vi "WPI_CANTalonSRX_Receive.vi"(11 "Device ID (0)":u8) -> (3 "Device ID":u8)   [LabVIEW 2016]
uses:
  <vilib>/Rock Robotics/WPI/ThirdParty/CanMotor/TalonSRX/WPI_CANTalonSRX_MessageIDs.ctl
  <vilib>/Rock Robotics/WPI/ThirdParty/CanMotor/TalonSRX/WPI_CANTalonSRX_GlobalOps.ctl
  <vilib>/Rock Robotics/WPI/ThirdParty/CanMotor/TalonSRX/WPI_CANTalonSRX_GlobalStatus.ctl
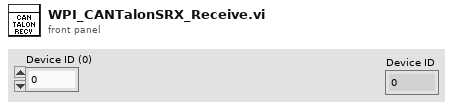
[diagram p1: front panel]
types:
  T1 = typedef "WPI_CANTalonSRX_MessageIDs.ctl" = u32
  T2 = typedef "WPI_CANTalonSRX_GlobalStatus.ctl" = cluster{"Applied Throttle":dbl, "Module Enabled":bool, "CAN Error":errorcluster, "Closed Loop Error":dbl, "Forward Limit Switch Closed":bool, "Reverse Limit Switch Closed":bool, "Sensor Position":dbl, "Sensor Velocity":dbl, "Current":dbl, "Sticky Fault - Over Temp":bool, "Sticky Fault - Under Voltage":bool, "Sticky Fault - Forward Limit":bool, "Sticky Fault - Reverse Limit":bool, "Sticky Fault - Forward Soft Limit":bool, "Sticky Fault - Reverse Soft Limit":bool, "Brake is Enabled":bool, "Encoder Position":dbl, "Encoder Velocity":dbl, "Encoder Index Count":dbl, "Encoder A Pin State":bool, "Encoder B Pin State":bool, "Encoder Index Pin State":bool, "Analog In":dbl, "Analog In Velocity":dbl, "Temperature (C)":dbl, "Battery Voltage":dbl, "Control 5 Is Supported":bool, "Current Profile Slot Select":dbl, "Pos Div 8":bool, "Vel Div 4":bool, "Pulse Width Position":i32, "Pulse Width Velocity":i32, "Pulse Width Rise To Rise (us)":i32, "Pulse Width Rise To Fall (us)":i32, "Mot Prof Active Is Under Run":bool, "Mot Prof Active Has Under Run":bool, "Mot Prof Active Is Last":bool, "Mot Prof Active Velocity Only":bool, "Mot Prof Active Is Valid":bool, "Mot Prof Buffer Is Full":bool, "Mot Prof Active Profile Slot Select":i32, "Mot Prof NextID":i32, "Mot Prof Count":i32, "Mot Prof Active Velocity":dbl, "Mot Prof Active Position":dbl, "Mot Prof Output Enable":i32}
  T3 = typedef "WPI_CANTalonSRX_GlobalOps.ctl" = enum16{"Read For Send", "Write After Receive General", "Write After Receive Feedback", "Write After Receive Encoder", "Write After Receive Ain", "Write Error", "Get All", "Set Output", "Set Mode", "Set Master ID", "Set Brake Mode", "Set Reverse Feedback Sensor", "Set Reverse Closed Loop Output", "Set Override Limits", "Set Forward Limit Enabled", "Set Reverse Limit Enabled", "Set Feedback Select", "Set Profile Select", "Set Throttle Ramp Rate", "Disable", "Set Enc Codes Per Rev", "Set Num Pot Turns", "Set Control Frame Rate", "Enable Legacy Control", "Write After Receive Pulse Width", "Set Enable Frame Rate", "Write After Receive Motion Profile", "Set Motion Profile Flow Control", "Set Motion Profile Control Frame Rate", "Set Current Limit Enable"}
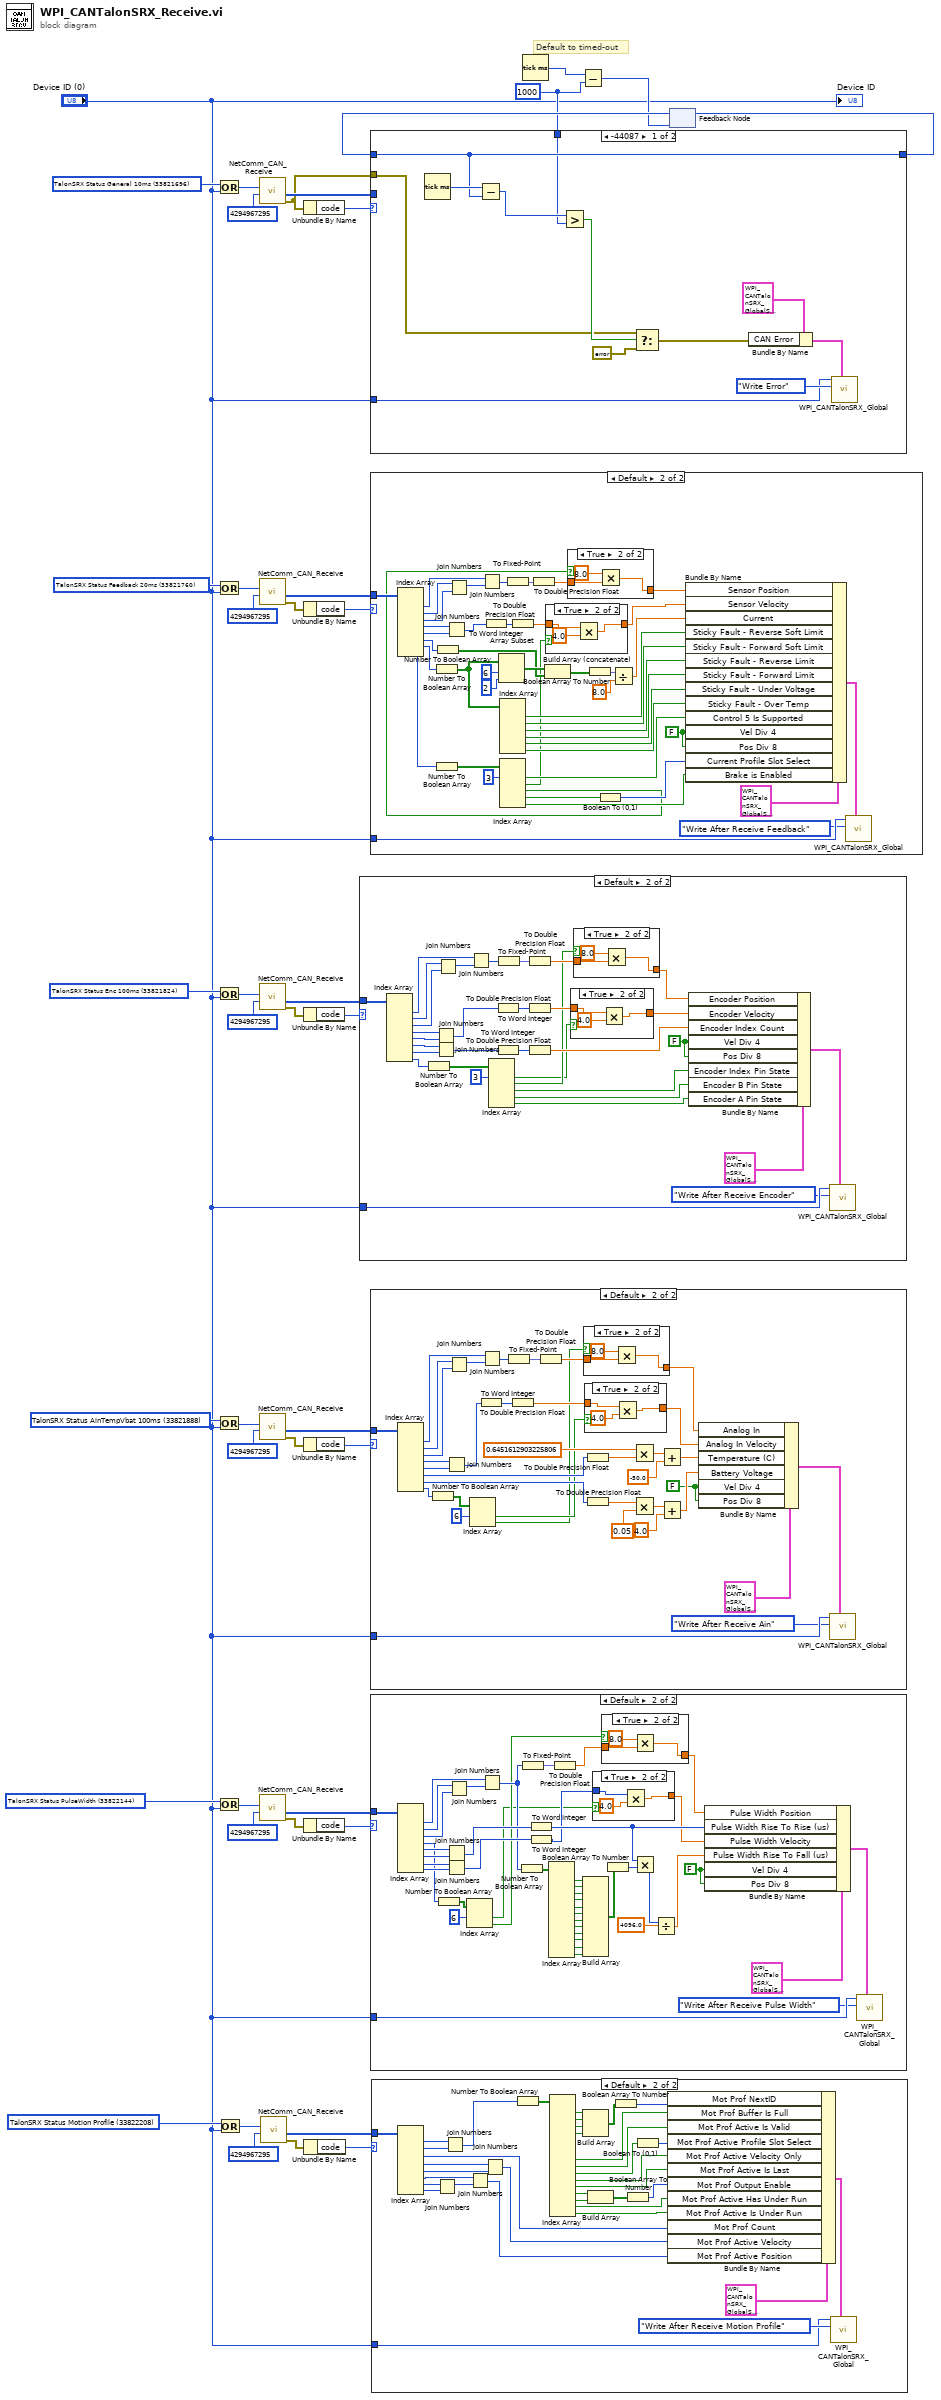
[diagram p0: block diagram]
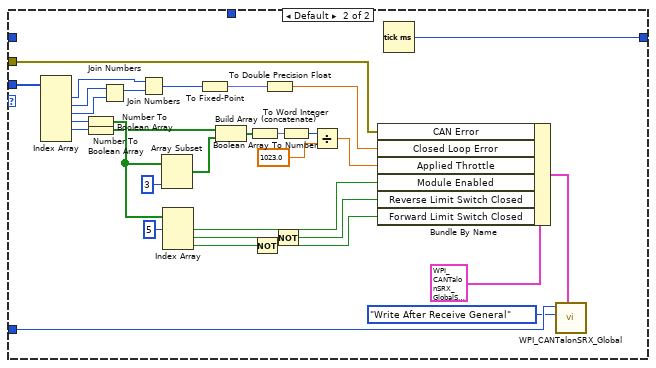
[diagram p15: hidden frame]
diagram:
  w2 = T1 33822208 items=["TalonSRX Control General 10ms"=33816576, "TalonSRX Control Rates Slow"=33816640, "TalonSRX Control ClearFlags Slow"=33816704, "TalonSRX Status General 10ms"=33821696, "TalonSRX Status Feedback 20ms"=33821760, "TalonSRX Status Enc 100ms"=33821824, "TalonSRX Status AinTempVbat 100ms"=33821888, "TalonSRX Status Startup Once"=33821952, "TalonSRX Status Debug"=33822080, "TalonSRX Config SetGainsSlot0 A"=33823808, "TalonSRX Config SetGainsSlot0 B"=33823872, "TalonSRX Config SetGainsSlot1 A"=33823936, "TalonSRX Config SetGainsSlot1 B"=33824000, "TalonSRX Config SetSoftLimits"=33824064, "TalonSRX Config WebControl"=33824128, "TalonSRX Param Request"=33822720, "TalonSRX Param Response"=33822784, "TalonSRX Param Set"=33822848, "TalonSRX Status PulseWidth"=33822144, "TalonSRX Status Motion Profile"=33822208, "TalonSRX Control General 5"=33816832, "TalonSRX Control Motion Profile Add"=33816896] ("Talon SRX Control Frame")
  w8 = T1 33822144 items=["TalonSRX Control General 10ms"=33816576, "TalonSRX Control Rates Slow"=33816640, "TalonSRX Control ClearFlags Slow"=33816704, "TalonSRX Status General 10ms"=33821696, "TalonSRX Status Feedback 20ms"=33821760, "TalonSRX Status Enc 100ms"=33821824, "TalonSRX Status AinTempVbat 100ms"=33821888, "TalonSRX Status Startup Once"=33821952, "TalonSRX Status Debug"=33822080, "TalonSRX Config SetGainsSlot0 A"=33823808, "TalonSRX Config SetGainsSlot0 B"=33823872, "TalonSRX Config SetGainsSlot1 A"=33823936, "TalonSRX Config SetGainsSlot1 B"=33824000, "TalonSRX Config SetSoftLimits"=33824064, "TalonSRX Config WebControl"=33824128, "TalonSRX Param Request"=33822720, "TalonSRX Param Response"=33822784, "TalonSRX Param Set"=33822848, "TalonSRX Status PulseWidth"=33822144, "TalonSRX Status Motion Profile"=33822208, "TalonSRX Control General 5"=33816832, "TalonSRX Control Motion Profile Add"=33816896] ("Talon SRX Control Frame")
  w15 = u32 1000 ("y")
  w21 = T1 33821888 items=["TalonSRX Control General 10ms"=33816576, "TalonSRX Control Rates Slow"=33816640, "TalonSRX Control ClearFlags Slow"=33816704, "TalonSRX Status General 10ms"=33821696, "TalonSRX Status Feedback 20ms"=33821760, "TalonSRX Status Enc 100ms"=33821824, "TalonSRX Status AinTempVbat 100ms"=33821888, "TalonSRX Status Startup Once"=33821952, "TalonSRX Status Debug"=33822080, "TalonSRX Config SetGainsSlot0 A"=33823808, "TalonSRX Config SetGainsSlot0 B"=33823872, "TalonSRX Config SetGainsSlot1 A"=33823936, "TalonSRX Config SetGainsSlot1 B"=33824000, "TalonSRX Config SetSoftLimits"=33824064, "TalonSRX Config WebControl"=33824128, "TalonSRX Param Request"=33822720, "TalonSRX Param Response"=33822784, "TalonSRX Param Set"=33822848]
  w28 = T1 33821824 items=["TalonSRX Control General 10ms"=33816576, "TalonSRX Control Rates Slow"=33816640, "TalonSRX Control ClearFlags Slow"=33816704, "TalonSRX Status General 10ms"=33821696, "TalonSRX Status Feedback 20ms"=33821760, "TalonSRX Status Enc 100ms"=33821824, "TalonSRX Status AinTempVbat 100ms"=33821888, "TalonSRX Status Startup Once"=33821952, "TalonSRX Status Debug"=33822080, "TalonSRX Config SetGainsSlot0 A"=33823808, "TalonSRX Config SetGainsSlot0 B"=33823872, "TalonSRX Config SetGainsSlot1 A"=33823936, "TalonSRX Config SetGainsSlot1 B"=33824000, "TalonSRX Config SetSoftLimits"=33824064, "TalonSRX Config WebControl"=33824128, "TalonSRX Param Request"=33822720, "TalonSRX Param Response"=33822784, "TalonSRX Param Set"=33822848]
  w33 = T1 33821760 items=["TalonSRX Control General 10ms"=33816576, "TalonSRX Control Rates Slow"=33816640, "TalonSRX Control ClearFlags Slow"=33816704, "TalonSRX Status General 10ms"=33821696, "TalonSRX Status Feedback 20ms"=33821760, "TalonSRX Status Enc 100ms"=33821824, "TalonSRX Status AinTempVbat 100ms"=33821888, "TalonSRX Status Startup Once"=33821952, "TalonSRX Status Debug"=33822080, "TalonSRX Config SetGainsSlot0 A"=33823808, "TalonSRX Config SetGainsSlot0 B"=33823872, "TalonSRX Config SetGainsSlot1 A"=33823936, "TalonSRX Config SetGainsSlot1 B"=33824000, "TalonSRX Config SetSoftLimits"=33824064, "TalonSRX Config WebControl"=33824128, "TalonSRX Param Request"=33822720, "TalonSRX Param Response"=33822784, "TalonSRX Param Set"=33822848]
  w40 = T1 33821696 items=["TalonSRX Control General 10ms"=33816576, "TalonSRX Control Rates Slow"=33816640, "TalonSRX Control ClearFlags Slow"=33816704, "TalonSRX Status General 10ms"=33821696, "TalonSRX Status Feedback 20ms"=33821760, "TalonSRX Status Enc 100ms"=33821824, "TalonSRX Status AinTempVbat 100ms"=33821888, "TalonSRX Status Startup Once"=33821952, "TalonSRX Status Debug"=33822080, "TalonSRX Config SetGainsSlot0 A"=33823808, "TalonSRX Config SetGainsSlot0 B"=33823872, "TalonSRX Config SetGainsSlot1 A"=33823936, "TalonSRX Config SetGainsSlot1 B"=33824000, "TalonSRX Config SetSoftLimits"=33824064, "TalonSRX Config WebControl"=33824128, "TalonSRX Param Request"=33822720, "TalonSRX Param Response"=33822784, "TalonSRX Param Set"=33822848]
  # "Default to timed-out"
  n1 = Or(x=w40, y="Device ID (0)") -> (x .or. y?=w41:T1)
  n2 = Or(x=w33, y="Device ID (0)") -> (x .or. y?=w32:T1)
  n3 = Or(x=w28, y="Device ID (0)") -> (x .or. y?=w29:T1)
  n4 = Or(x=w21, y="Device ID (0)") -> (x .or. y?=w20:T1)
  n5 = Or(x=w8, y="Device ID (0)") -> (x .or. y?=w12:T1)
  n6 = Or(x=w2, y="Device ID (0)") -> (x .or. y?=w6:T1)
  n7 = call <vilib>:"NetComm_CAN_Receive.vi"("Message ID Mask"=u32 4294967295, "Message ID"=w41) -> ("error out"=w38:errorcluster, "Data"=w42:u8[])  [unwired: 6 in, 2 out]
  n8 = call <vilib>:"NetComm_CAN_Receive.vi"("Message ID Mask"=u32 4294967295, "Message ID"=w32) -> ("error out"=w35:errorcluster, "Data"=w31:u8[])  [unwired: 6 in, 2 out]
  n9 = call <vilib>:"NetComm_CAN_Receive.vi"("Message ID Mask"=u32 4294967295, "Message ID"=w29) -> ("error out"=w26:errorcluster, "Data"=w30:u8[])  [unwired: 6 in, 2 out]
  n10 = call <vilib>:"NetComm_CAN_Receive.vi"("Message ID Mask"=u32 4294967295, "Message ID"=w20) -> ("error out"=w23:errorcluster, "Data"=w19:u8[])  [unwired: 6 in, 2 out]
  n11 = call <vilib>:"NetComm_CAN_Receive.vi"("Message ID Mask"=u32 4294967295, "Message ID"=w12) -> ("error out"=w10:errorcluster, "Data"=w13:u8[])  [unwired: 6 in, 2 out]
  n12 = call <vilib>:"NetComm_CAN_Receive.vi"("Message ID Mask"=u32 4294967295, "Message ID"=w6) -> ("error out"=w4:errorcluster, "Data"=w7:u8[])  [unwired: 6 in, 2 out]
  n13 = Unbundle By Name(w38) -> ("code"=w37:i32)
  n14 = Unbundle By Name(w35) -> ("code"=w36:i32)
  n15 = Unbundle By Name(w26) -> ("code"=w25:i32)
  n16 = Unbundle By Name(w23) -> ("code"=w24:i32)
  n17 = Unbundle By Name(w10) -> ("code"=w9:i32)
  n18 = Unbundle By Name(w4) -> ("code"=w3:i32)
  n19 = case shown="Default" w25 {
    tunnel: "Device ID (0)" -> [_ w75]
    tunnel: w30 -> [_ w74]
    frame -44087 {
    }
    frame Default {
      w43 = FALSE ("Vel Div 4")
      n20 = Index Array(array=w74) -> (element #1=w67:u8, element #2=w69:u8, element #3=w66:u8, element #4=w65:u8, element #5=w64:u8, element #6=w60:u8, element #7=w59:u8, element #8=w62:u8)  [unwired: 8 in]
      n21 = Number To Boolean Array(number=w62) -> (Boolean array=w72:bool[])
      n22 = Join Numbers(hi=w65, lo=w64) -> ((hi.lo)=w63:u16)
      n23 = Join Numbers(hi=w60, lo=w59) -> ((hi.lo)=w56:u16)
      n24 = Join Numbers(hi=w69, lo=w66) -> ((hi.lo)=w68:u16)
      n25 = Join Numbers(hi=w67, lo=w68) -> ((hi.lo)=w54:u32)
      n26 = Index Array(array=w72, index #1=3 ("index")) -> (element #1=w44:bool, element #2=w45:bool, element #3=w46:bool, element #4=w47:bool, element #5=w48:bool)  [unwired: 4 in]
      n27 = To Word Integer(number=w63) -> (16bit integer=w57:i16)
      n28 = To Word Integer(number=w56) -> (16bit integer=w55:i16)
      n29 = To Fixed-Point(number=w54) -> (fixed-point=w53:fxp<+/-,24,24>)  [unwired: 1 in]
      n30 = To Double Precision Float(number=w53) -> (double precision float=w51:dbl)
      n31 = To Double Precision Float(number=w57) -> (double precision float=w52:dbl)
      n32 = To Double Precision Float(number=w55) -> (double precision float=w61:dbl)
      n33 = case shown="True" w44 {
        tunnel: w52 -> [w76 w79]
        tunnel: [w76 w77] -> w50
        frame False {
        }
        frame True {
          n34 = Multiply(x=w79, y=4.0) -> (x*y=w77:dbl)
        }
      }
      n35 = case shown="True" w45 {
        tunnel: w51 -> [w80 w83]
        tunnel: [w80 w81] -> w49
        frame False {
        }
        frame True {
          n36 = Multiply(x=8.0, y=w83) -> (x*y=w81:dbl)
        }
      }
      n37 = Bundle By Name(cluster=T2 {"Applied Throttle"=0.0, "Module Enabled"=FALSE, "CAN Error"={"status"=FALSE, "code"=0, "source"=""}, "Closed Loop Error"=0.0, "Forward Limit Switch Closed"=FALSE, "Reverse Limit Switch Closed"=FALSE, "Sensor Position"=0.0, "Sensor Velocity"=0.0, "Current"=0.0, "Sticky Fault - Over Temp"=FALSE, "Sticky Fault - Under Voltage"=FALSE, "Sticky Fault - Forward Limit"=FALSE, "Sticky Fault - Reverse Limit"=FALSE, "Sticky Fault - Forward Soft Limit"=FALSE, "Sticky Fault - Reverse Soft Limit"=FALSE, "Brake is Enabled"=FALSE, "Encoder Position"=0.0, "Encoder Velocity"=0.0, "Encoder Index Count"=0.0, "Encoder A Pin State"=FALSE, "Encoder B Pin State"=FALSE, "Encoder Index Pin State"=FALSE, "Analog In"=0.0, "Analog In Velocity"=0.0, "Temperature (C)"=0.0, "Battery Voltage"=0.0, "Control 5 Is Supported"=FALSE, "Current Profile Slot Select"=0.0, "Pos Div 8"=FALSE, "Vel Div 4"=FALSE, "Pulse Width Position"=0, "Pulse Width Velocity"=0, "Pulse Width Rise To Rise (us)"=0, "Pulse Width Rise To Fall (us)"=0, "Mot Prof Active Is Under Run"=FALSE, "Mot Prof Active Has Under Run"=FALSE, "Mot Prof Active Is Last"=FALSE, "Mot Prof Active Velocity Only"=FALSE, "Mot Prof Active Is Valid"=FALSE, "Mot Prof Buffer Is Full"=FALSE, "Mot Prof Active Profile Slot Select"=0, "Mot Prof NextID"=0, "Mot Prof Count"=0, "Mot Prof Active Velocity"=0.0, "Mot Prof Active Position"=0.0, "Mot Prof Output Enable"=0} ("Write After Receive"), "Encoder Position"=w49, "Encoder Velocity"=w50, "Encoder Index Count"=w61, "Vel Div 4"=w43, "Pos Div 8"=w43, "Encoder Index Pin State"=w46, "Encoder B Pin State"=w47, "Encoder A Pin State"=w48) -> (w73:T2)
      n38 = call <vilib>:"WPI_CANTalonSRX_Global.vi"("Write After Receive"=w73, "Operation"=WPI_CANTalonSRX_GlobalOps."Write After Receive Encoder", "Device ID (0)"=w75) -> ()  [unwired: 6 in, 3 out]
    }
  }
  n39 = case shown="Default" w36 {
    tunnel: "Device ID (0)" -> [_ w129]
    tunnel: w31 -> [_ w128]
    frame -44087 {
    }
    frame Default {
      w84 = FALSE ("Vel Div 4")
      n40 = Index Array(array=w128) -> (element #1=w117:u8, element #2=w119:u8, element #3=w116:u8, element #4=w115:u8, element #5=w114:u8, element #6=w112:u8, element #7=w111:u8, element #8=w107:u8)  [unwired: 8 in]
      n41 = Number To Boolean Array(number=w111) -> (Boolean array=w126:bool[])
      n42 = Number To Boolean Array(number=w107) -> (Boolean array=w106:bool[])
      n43 = Number To Boolean Array(number=w112) -> (Boolean array=w97:bool[])
      n44 = Join Numbers(hi=w115, lo=w114) -> ((hi.lo)=w113:u16)
      n45 = Join Numbers(hi=w119, lo=w116) -> ((hi.lo)=w118:u16)
      n46 = Join Numbers(hi=w117, lo=w118) -> ((hi.lo)=w96:u32)
      n47 = To Word Integer(number=w113) -> (16bit integer=w99:i16)
      n48 = Array Subset(array=w126, index=6, length=2) -> (w98:bool[])
      n49 = Index Array(array=w126) -> (element #1=w104:bool, element #2=w103:bool, element #3=w102:bool, element #4=w101:bool, element #5=w100:bool, element #6=w105:bool)  [unwired: 6 in]
      n50 = Index Array(array=w106, index #1=3 ("index")) -> (element #1=w93:bool, element #2=w85:bool, element #3=w88:bool, element #4=w91:bool, element #5=w94:bool)  [unwired: 4 in]
      n51 = To Fixed-Point(number=w96) -> (fixed-point=w95:fxp<+/-,24,24>)  [unwired: 1 in]
      n52 = To Double Precision Float(number=w99) -> (double precision float=w87:dbl)
      n53 = To Double Precision Float(number=w95) -> (double precision float=w90:dbl)
      n54 = Build Array (concatenate)(w98, w97) -> (w124:bool[])
      n55 = case shown="True" w85 {
        tunnel: w87 -> [w130 w133]
        tunnel: [w130 w131] -> w86
        frame False {
        }
        frame True {
          n56 = Multiply(x=w133, y=4.0) -> (x*y=w131:dbl)
        }
      }
      n57 = case shown="True" w88 {
        tunnel: w90 -> [w134 w137]
        tunnel: [w134 w135] -> w89
        frame False {
        }
        frame True {
          n58 = Multiply(x=8.0, y=w137) -> (x*y=w135:dbl)
        }
      }
      n59 = Boolean Array To Number(Boolean array=w124) -> (number=w123:fxp<+/-,11,11>)
      n60 = Boolean To (0,1)(Boolean=w91) -> (0, 1=w92:i16)
      n61 = Divide(x=w123, y=8.0) -> (x/y=w109:dbl)
      n62 = Bundle By Name(cluster=T2 {"Applied Throttle"=0.0, "Module Enabled"=FALSE, "CAN Error"={"status"=FALSE, "code"=0, "source"=""}, "Closed Loop Error"=0.0, "Forward Limit Switch Closed"=FALSE, "Reverse Limit Switch Closed"=FALSE, "Sensor Position"=0.0, "Sensor Velocity"=0.0, "Current"=0.0, "Sticky Fault - Over Temp"=FALSE, "Sticky Fault - Under Voltage"=FALSE, "Sticky Fault - Forward Limit"=FALSE, "Sticky Fault - Reverse Limit"=FALSE, "Sticky Fault - Forward Soft Limit"=FALSE, "Sticky Fault - Reverse Soft Limit"=FALSE, "Brake is Enabled"=FALSE, "Encoder Position"=0.0, "Encoder Velocity"=0.0, "Encoder Index Count"=0.0, "Encoder A Pin State"=FALSE, "Encoder B Pin State"=FALSE, "Encoder Index Pin State"=FALSE, "Analog In"=0.0, "Analog In Velocity"=0.0, "Temperature (C)"=0.0, "Battery Voltage"=0.0, "Control 5 Is Supported"=FALSE, "Current Profile Slot Select"=0.0, "Pos Div 8"=FALSE, "Vel Div 4"=FALSE, "Pulse Width Position"=0, "Pulse Width Velocity"=0, "Pulse Width Rise To Rise (us)"=0, "Pulse Width Rise To Fall (us)"=0, "Mot Prof Active Is Under Run"=FALSE, "Mot Prof Active Has Under Run"=FALSE, "Mot Prof Active Is Last"=FALSE, "Mot Prof Active Velocity Only"=FALSE, "Mot Prof Active Is Valid"=FALSE, "Mot Prof Buffer Is Full"=FALSE, "Mot Prof Active Profile Slot Select"=0, "Mot Prof NextID"=0, "Mot Prof Count"=0, "Mot Prof Active Velocity"=0.0, "Mot Prof Active Position"=0.0, "Mot Prof Output Enable"=0} ("Write After Receive"), "Sensor Position"=w89, "Sensor Velocity"=w86, "Current"=w109, "Sticky Fault - Reverse Soft Limit"=w104, "Sticky Fault - Forward Soft Limit"=w103, "Sticky Fault - Reverse Limit"=w102, "Sticky Fault - Forward Limit"=w101, "Sticky Fault - Under Voltage"=w100, "Sticky Fault - Over Temp"=w105, "Control 5 Is Supported"=w93, "Vel Div 4"=w84, "Pos Div 8"=w84, "Current Profile Slot Select"=w92, "Brake is Enabled"=w94) -> (w127:T2)
      n63 = call <vilib>:"WPI_CANTalonSRX_Global.vi"("Write After Receive"=w127, "Operation"=WPI_CANTalonSRX_GlobalOps."Write After Receive Feedback", "Device ID (0)"=w129) -> ()  [unwired: 6 in, 3 out]
    }
  }
  n64 = case shown="Default" w24 {
    tunnel: "Device ID (0)" -> [_ w174]
    tunnel: w19 -> [_ w173]
    frame -44087 {
    }
    frame Default {
      w138 = FALSE ("Vel Div 4")
      n65 = Index Array(array=w173) -> (element #1=w167:u8, element #2=w169:u8, element #3=w166:u8, element #4=w165:u8, element #5=w164:u8, element #6=w160:u8, element #7=w161:u8, element #8=w147:u8)  [unwired: 8 in]
      n66 = Number To Boolean Array(number=w147) -> (Boolean array=w146:bool[])
      n67 = Join Numbers(hi=w165, lo=w164) -> ((hi.lo)=w163:u16)
      n68 = Join Numbers(hi=w169, lo=w166) -> ((hi.lo)=w168:u16)
      n69 = Index Array(array=w146, index #1=6 ("index")) -> (element #1=w140:bool, element #2=w139:bool)  [unwired: 1 in]
      n70 = To Word Integer(number=w163) -> (16bit integer=w150:i16)
      n71 = Join Numbers(hi=w167, lo=w168) -> ((hi.lo)=w149:u32)
      n72 = To Fixed-Point(number=w149) -> (fixed-point=w148:fxp<+/-,24,24>)  [unwired: 1 in]
      n73 = To Double Precision Float(number=w150) -> (double precision float=w142:dbl)
      n74 = To Double Precision Float(number=w148) -> (double precision float=w144:dbl)
      n75 = case shown="True" w139 {
        tunnel: w144 -> [w179 w182]
        tunnel: [w179 w180] -> w143
        frame False {
        }
        frame True {
          n76 = Multiply(x=8.0, y=w182) -> (x*y=w180:dbl)
        }
      }
      n77 = case shown="True" w140 {
        tunnel: w142 -> [w175 w178]
        tunnel: [w175 w176] -> w141
        frame False {
        }
        frame True {
          n78 = Multiply(x=w178, y=4.0) -> (x*y=w176:dbl)
        }
      }
      n79 = To Double Precision Float(number=w160) -> (double precision float=w151:dbl)
      n80 = To Double Precision Float(number=w161) -> (double precision float=w162:dbl)
      n81 = Multiply(x=0.6451612903225806, y=w151) -> (x*y=w155:dbl)
      n82 = Multiply(x=w162, y=0.05 ("x")) -> (x*y=w157:dbl)
      n83 = Add(x=w155, y=-50.0 ("x")) -> (x+y=w153:dbl)
      n84 = Add(x=w157, y=4.0 ("x")) -> (x+y=w159:dbl)
      n85 = Bundle By Name(cluster=T2 {"Applied Throttle"=0.0, "Module Enabled"=FALSE, "CAN Error"={"status"=FALSE, "code"=0, "source"=""}, "Closed Loop Error"=0.0, "Forward Limit Switch Closed"=FALSE, "Reverse Limit Switch Closed"=FALSE, "Sensor Position"=0.0, "Sensor Velocity"=0.0, "Current"=0.0, "Sticky Fault - Over Temp"=FALSE, "Sticky Fault - Under Voltage"=FALSE, "Sticky Fault - Forward Limit"=FALSE, "Sticky Fault - Reverse Limit"=FALSE, "Sticky Fault - Forward Soft Limit"=FALSE, "Sticky Fault - Reverse Soft Limit"=FALSE, "Brake is Enabled"=FALSE, "Encoder Position"=0.0, "Encoder Velocity"=0.0, "Encoder Index Count"=0.0, "Encoder A Pin State"=FALSE, "Encoder B Pin State"=FALSE, "Encoder Index Pin State"=FALSE, "Analog In"=0.0, "Analog In Velocity"=0.0, "Temperature (C)"=0.0, "Battery Voltage"=0.0, "Control 5 Is Supported"=FALSE, "Current Profile Slot Select"=0.0, "Pos Div 8"=FALSE, "Vel Div 4"=FALSE, "Pulse Width Position"=0, "Pulse Width Velocity"=0, "Pulse Width Rise To Rise (us)"=0, "Pulse Width Rise To Fall (us)"=0, "Mot Prof Active Is Under Run"=FALSE, "Mot Prof Active Has Under Run"=FALSE, "Mot Prof Active Is Last"=FALSE, "Mot Prof Active Velocity Only"=FALSE, "Mot Prof Active Is Valid"=FALSE, "Mot Prof Buffer Is Full"=FALSE, "Mot Prof Active Profile Slot Select"=0, "Mot Prof NextID"=0, "Mot Prof Count"=0, "Mot Prof Active Velocity"=0.0, "Mot Prof Active Position"=0.0, "Mot Prof Output Enable"=0} ("Write After Receive"), "Analog In"=w143, "Analog In Velocity"=w141, "Temperature (C)"=w153, "Battery Voltage"=w159, "Vel Div 4"=w138, "Pos Div 8"=w138) -> (w172:T2)
      n86 = call <vilib>:"WPI_CANTalonSRX_Global.vi"("Write After Receive"=w172, "Operation"=WPI_CANTalonSRX_GlobalOps."Write After Receive Ain", "Device ID (0)"=w174) -> ()  [unwired: 6 in, 3 out]
    }
  }
  n87 = case shown="Default" w9 {
    tunnel: "Device ID (0)" -> [_ w228]
    tunnel: w13 -> [_ w227]
    frame -44087 {
    }
    frame Default {
      w183 = FALSE ("Vel Div 4")
      n88 = Index Array(array=w227) -> (element #1=w221:u8, element #2=w223:u8, element #3=w220:u8, element #4=w192:u8, element #5=w216:u8, element #6=w215:u8, element #7=w214:u8, element #8=w213:u8)  [unwired: 8 in]
      n89 = Number To Boolean Array(number=w192) -> (Boolean array=w191:bool[])
      n90 = Join Numbers(hi=w216, lo=w215) -> ((hi.lo)=w219:u16)
      n91 = Join Numbers(hi=w214, lo=w213) -> ((hi.lo)=w218:u16)
      n92 = Join Numbers(hi=w223, lo=w220) -> ((hi.lo)=w222:u16)
      n93 = Index Array(array=w191, index #1=6 ("index")) -> (element #1=w184:bool, element #2=w185:bool)  [unwired: 1 in]
      n94 = Join Numbers(hi=w221, lo=w222) -> ((hi.lo)=w193:u32)
      n95 = Number To Boolean Array(number=w193) -> (Boolean array=w208:bool[])
      n96 = To Fixed-Point(number=w193) -> (fixed-point=w217:fxp<+/-,24,24>)  [unwired: 1 in]
      n97 = To Word Integer(number=w219) -> (16bit integer=w209:i16)
      n98 = To Word Integer(number=w218) -> (16bit integer=w187:i16)
      n99 = Index Array(array=w208) -> (element #1=w198:bool, element #2=w199:bool, element #3=w200:bool, element #4=w201:bool, element #5=w202:bool, element #6=w203:bool, element #7=w204:bool, element #8=w205:bool, element #9=w206:bool, element #10=w207:bool, element #11=w195:bool, element #12=w194:bool)  [unwired: 12 in]
      n100 = To Double Precision Float(number=w217) -> (double precision float=w188:dbl)
      n101 = Build Array(w198, w199, w200, w201, w202, w203, w204, w205, w206, w207, w195, w194) -> (w197:bool[])
      n102 = case shown="True" w184 {
        tunnel: w187 -> [w229 w232]
        tunnel: [w229 w230] -> w186
        frame False {
        }
        frame True {
          n103 = Multiply(x=w232, y=4.0) -> (x*y=w230:dbl)
        }
      }
      n104 = case shown="True" w185 {
        tunnel: w188 -> [w233 w236]
        tunnel: [w233 w234] -> w189
        frame False {
        }
        frame True {
          n105 = Multiply(x=8.0, y=w236) -> (x*y=w234:dbl)
        }
      }
      n106 = Boolean Array To Number(Boolean array=w197) -> (number=w196:u32)
      n107 = Multiply(x=w209, y=w196) -> (x*y=w211:u32)
      n108 = Divide(x=w211, y=4096.0) -> (x/y=w210:dbl)
      n109 = Bundle By Name(cluster=T2 {"Applied Throttle"=0.0, "Module Enabled"=FALSE, "CAN Error"={"status"=FALSE, "code"=0, "source"=""}, "Closed Loop Error"=0.0, "Forward Limit Switch Closed"=FALSE, "Reverse Limit Switch Closed"=FALSE, "Sensor Position"=0.0, "Sensor Velocity"=0.0, "Current"=0.0, "Sticky Fault - Over Temp"=FALSE, "Sticky Fault - Under Voltage"=FALSE, "Sticky Fault - Forward Limit"=FALSE, "Sticky Fault - Reverse Limit"=FALSE, "Sticky Fault - Forward Soft Limit"=FALSE, "Sticky Fault - Reverse Soft Limit"=FALSE, "Brake is Enabled"=FALSE, "Encoder Position"=0.0, "Encoder Velocity"=0.0, "Encoder Index Count"=0.0, "Encoder A Pin State"=FALSE, "Encoder B Pin State"=FALSE, "Encoder Index Pin State"=FALSE, "Analog In"=0.0, "Analog In Velocity"=0.0, "Temperature (C)"=0.0, "Battery Voltage"=0.0, "Control 5 Is Supported"=FALSE, "Current Profile Slot Select"=0.0, "Pos Div 8"=FALSE, "Vel Div 4"=FALSE, "Pulse Width Position"=0, "Pulse Width Velocity"=0, "Pulse Width Rise To Rise (us)"=0, "Pulse Width Rise To Fall (us)"=0, "Mot Prof Active Is Under Run"=FALSE, "Mot Prof Active Has Under Run"=FALSE, "Mot Prof Active Is Last"=FALSE, "Mot Prof Active Velocity Only"=FALSE, "Mot Prof Active Is Valid"=FALSE, "Mot Prof Buffer Is Full"=FALSE, "Mot Prof Active Profile Slot Select"=0, "Mot Prof NextID"=0, "Mot Prof Count"=0, "Mot Prof Active Velocity"=0.0, "Mot Prof Active Position"=0.0, "Mot Prof Output Enable"=0} ("Write After Receive"), "Pulse Width Position"=w189, "Pulse Width Rise To Rise (us)"=w209, "Pulse Width Velocity"=w186, "Pulse Width Rise To Fall (us)"=w210, "Vel Div 4"=w183, "Pos Div 8"=w183) -> (w226:T2)
      n110 = call <vilib>:"WPI_CANTalonSRX_Global.vi"("Write After Receive"=w226, "Operation"=WPI_CANTalonSRX_GlobalOps."Write After Receive Pulse Width", "Device ID (0)"=w228) -> ()  [unwired: 6 in, 3 out]
    }
  }
  n111 = case shown="Default" w3 {
    tunnel: w7 -> [_ w272]
    tunnel: "Device ID (0)" -> [_ w267]
    frame -44087 {
    }
    frame Default {
      n112 = Index Array(array=w272) -> (element #1=w260:u8, element #2=w259:u8, element #3=w237:u8, element #4=w262:u8, element #5=w263:u8, element #6=w266:u8, element #7=w265:u8, element #8=w264:u8)  [unwired: 8 in]
      n113 = Join Numbers(hi=w265, lo=w264) -> ((hi.lo)=w268:u16)
      n114 = Join Numbers(hi=w260, lo=w259) -> ((hi.lo)=w258:u16)
      n115 = Join Numbers(hi=w266, lo=w268) -> ((hi.lo)=w239:u32)
      n116 = Join Numbers(hi=w262, lo=w263) -> ((hi.lo)=w238:u16)
      n117 = Number To Boolean Array(number=w258) -> (Boolean array=w261:bool[])
      n118 = Index Array(array=w261) -> (element #1=w257:bool, element #2=w256:bool, element #3=w255:bool, element #4=w254:bool, element #8=w251:bool, element #9=w250:bool, element #10=w240:bool, element #11=w249:bool, element #12=w248:bool, element #13=w245:bool, element #14=w244:bool, element #15=w246:bool, element #16=w247:bool)  [unwired: 16 in, 3 out]
      n119 = Build Array(w257, w256, w255, w254) -> (w253:bool[])
      n120 = Build Array(w245, w244) -> (w242:bool[])
      n121 = Boolean Array To Number(Boolean array=w253) -> (number=w252:u32)
      n122 = Boolean Array To Number(Boolean array=w242) -> (number=w243:u32)
      n123 = Boolean To (0,1)(Boolean=w240) -> (0, 1=w241:i16)
      n124 = Bundle By Name(cluster=T2 {"Applied Throttle"=0.0, "Module Enabled"=FALSE, "CAN Error"={"status"=FALSE, "code"=0, "source"=""}, "Closed Loop Error"=0.0, "Forward Limit Switch Closed"=FALSE, "Reverse Limit Switch Closed"=FALSE, "Sensor Position"=0.0, "Sensor Velocity"=0.0, "Current"=0.0, "Sticky Fault - Over Temp"=FALSE, "Sticky Fault - Under Voltage"=FALSE, "Sticky Fault - Forward Limit"=FALSE, "Sticky Fault - Reverse Limit"=FALSE, "Sticky Fault - Forward Soft Limit"=FALSE, "Sticky Fault - Reverse Soft Limit"=FALSE, "Brake is Enabled"=FALSE, "Encoder Position"=0.0, "Encoder Velocity"=0.0, "Encoder Index Count"=0.0, "Encoder A Pin State"=FALSE, "Encoder B Pin State"=FALSE, "Encoder Index Pin State"=FALSE, "Analog In"=0.0, "Analog In Velocity"=0.0, "Temperature (C)"=0.0, "Battery Voltage"=0.0, "Control 5 Is Supported"=FALSE, "Current Profile Slot Select"=0.0, "Pos Div 8"=FALSE, "Vel Div 4"=FALSE, "Pulse Width Position"=0, "Pulse Width Velocity"=0, "Pulse Width Rise To Rise (us)"=0, "Pulse Width Rise To Fall (us)"=0, "Mot Prof Active Is Under Run"=FALSE, "Mot Prof Active Has Under Run"=FALSE, "Mot Prof Active Is Last"=FALSE, "Mot Prof Active Velocity Only"=FALSE, "Mot Prof Active Is Valid"=FALSE, "Mot Prof Buffer Is Full"=FALSE, "Mot Prof Active Profile Slot Select"=0, "Mot Prof NextID"=0, "Mot Prof Count"=0, "Mot Prof Active Velocity"=0.0, "Mot Prof Active Position"=0.0, "Mot Prof Output Enable"=0} ("Write After Receive"), "Mot Prof NextID"=w252, "Mot Prof Buffer Is Full"=w251, "Mot Prof Active Is Valid"=w250, "Mot Prof Active Profile Slot Select"=w241, "Mot Prof Active Velocity Only"=w249, "Mot Prof Active Is Last"=w248, "Mot Prof Output Enable"=w243, "Mot Prof Active Has Under Run"=w246, "Mot Prof Active Is Under Run"=w247, "Mot Prof Count"=w237, "Mot Prof Active Velocity"=w238, "Mot Prof Active Position"=w239) -> (w271:T2)
      n125 = call <vilib>:"WPI_CANTalonSRX_Global.vi"("Write After Receive"=w271, "Operation"=WPI_CANTalonSRX_GlobalOps."Write After Receive Motion Profile", "Device ID (0)"=w267) -> ()  [unwired: 6 in, 3 out]
    }
  }
  n126 = Tick Count (ms)() -> (millisecond timer value=w16:u32)
  n127 = Subtract(x=w16, y=w15) -> (x-y=w14:u32)
  n128 = feedback #1(w14) -> (w17:u32)
  n129 = case shown="-44087" w37 {
    tunnel: "Device ID (0)" -> [w283 w315]
    tunnel: w42 -> [_ w314]
    tunnel: w38 -> [w276 w288]
    tunnel: [w279 w287] -> w18
    tunnel: w17 -> [w279 _]
    tunnel: w15 -> [w273 _]
    frame -44087 {
      n130 = Tick Count (ms)() -> (millisecond timer value=w280:u32)
      n131 = Subtract(x=w280, y=w279) -> (x-y=w278:u32)
      n132 = Greater?(x=w278, y=w273) -> (0:w277:bool)
      n133 = Select(t=w276, s=w277, f=errorcluster {"status"=FALSE, "code"=0, "source"=""}) -> (s? t:f=w275:errorcluster)
      n134 = Bundle By Name(cluster=T2 {"Applied Throttle"=0.0, "Module Enabled"=FALSE, "CAN Error"={"status"=FALSE, "code"=0, "source"=""}, "Closed Loop Error"=0.0, "Forward Limit Switch Closed"=FALSE, "Reverse Limit Switch Closed"=FALSE, "Sensor Position"=0.0, "Sensor Velocity"=0.0, "Current"=0.0, "Sticky Fault - Over Temp"=FALSE, "Sticky Fault - Under Voltage"=FALSE, "Sticky Fault - Forward Limit"=FALSE, "Sticky Fault - Reverse Limit"=FALSE, "Sticky Fault - Forward Soft Limit"=FALSE, "Sticky Fault - Reverse Soft Limit"=FALSE, "Brake is Enabled"=FALSE, "Encoder Position"=0.0, "Encoder Velocity"=0.0, "Encoder Index Count"=0.0, "Encoder A Pin State"=FALSE, "Encoder B Pin State"=FALSE, "Encoder Index Pin State"=FALSE, "Analog In"=0.0, "Analog In Velocity"=0.0, "Temperature (C)"=0.0, "Battery Voltage"=0.0, "Control 5 Is Supported"=FALSE, "Current Profile Slot Select"=0.0, "Pos Div 8"=FALSE, "Vel Div 4"=FALSE, "Pulse Width Position"=0, "Pulse Width Velocity"=0, "Pulse Width Rise To Rise (us)"=0, "Pulse Width Rise To Fall (us)"=0, "Mot Prof Active Is Under Run"=FALSE, "Mot Prof Active Has Under Run"=FALSE, "Mot Prof Active Is Last"=FALSE, "Mot Prof Active Velocity Only"=FALSE, "Mot Prof Active Is Valid"=FALSE, "Mot Prof Buffer Is Full"=FALSE, "Mot Prof Active Profile Slot Select"=0, "Mot Prof NextID"=0, "Mot Prof Count"=0, "Mot Prof Active Velocity"=0.0, "Mot Prof Active Position"=0.0, "Mot Prof Output Enable"=0} ("Write After Receive"), "CAN Error"=w275) -> (w281:T2)
      n135 = call <vilib>:"WPI_CANTalonSRX_Global.vi"("Write After Receive"=w281, "Operation"=WPI_CANTalonSRX_GlobalOps."Write Error", "Device ID (0)"=w283) -> ()  [unwired: 6 in, 3 out]
    }
    frame Default {
      n136 = Index Array(array=w314) -> (element #1=w295:u8, element #2=w298:u8, element #3=w294:u8, element #4=w310:u8, element #5=w307:u8)  [unwired: 6 in, 1 out]
      n137 = Number To Boolean Array(number=w310) -> (Boolean array=w309:bool[])
      n138 = Number To Boolean Array(number=w307) -> (Boolean array=w306:bool[])
      n139 = Join Numbers(hi=w298, lo=w294) -> ((hi.lo)=w297:u16)
      n140 = Join Numbers(hi=w295, lo=w297) -> ((hi.lo)=w296:u32)
      n141 = Array Subset(array=w309, length=3) -> (w305:bool[])  [unwired: 1 in]
      n142 = Index Array(array=w309, index #1=5 ("index")) -> (element #1=w311:bool, element #2=w290:bool, element #3=w289:bool)  [unwired: 2 in]
      n143 = To Fixed-Point(number=w296) -> (fixed-point=w292:fxp<+/-,24,24>)  [unwired: 1 in]
      n144 = Build Array (concatenate)(w306, w305) -> (w304:bool[])
      n145 = Boolean Array To Number(Boolean array=w304) -> (number=w303:fxp<+/-,11,11>)
      n146 = Not(x=w289) -> (.not. x?=w286:bool)
      n147 = To Double Precision Float(number=w292) -> (double precision float=w293:dbl)
      n148 = Not(x=w290) -> (.not. x?=w285:bool)
      n149 = To Word Integer(number=w303) -> (16bit integer=w291:i16)
      n150 = Divide(x=w291, y=1023.0) -> (x/y=w301:dbl)
      n151 = Bundle By Name(cluster=T2 {"Applied Throttle"=0.0, "Module Enabled"=FALSE, "CAN Error"={"status"=FALSE, "code"=0, "source"=""}, "Closed Loop Error"=0.0, "Forward Limit Switch Closed"=FALSE, "Reverse Limit Switch Closed"=FALSE, "Sensor Position"=0.0, "Sensor Velocity"=0.0, "Current"=0.0, "Sticky Fault - Over Temp"=FALSE, "Sticky Fault - Under Voltage"=FALSE, "Sticky Fault - Forward Limit"=FALSE, "Sticky Fault - Reverse Limit"=FALSE, "Sticky Fault - Forward Soft Limit"=FALSE, "Sticky Fault - Reverse Soft Limit"=FALSE, "Brake is Enabled"=FALSE, "Encoder Position"=0.0, "Encoder Velocity"=0.0, "Encoder Index Count"=0.0, "Encoder A Pin State"=FALSE, "Encoder B Pin State"=FALSE, "Encoder Index Pin State"=FALSE, "Analog In"=0.0, "Analog In Velocity"=0.0, "Temperature (C)"=0.0, "Battery Voltage"=0.0, "Control 5 Is Supported"=FALSE, "Current Profile Slot Select"=0.0, "Pos Div 8"=FALSE, "Vel Div 4"=FALSE, "Pulse Width Position"=0, "Pulse Width Velocity"=0, "Pulse Width Rise To Rise (us)"=0, "Pulse Width Rise To Fall (us)"=0, "Mot Prof Active Is Under Run"=FALSE, "Mot Prof Active Has Under Run"=FALSE, "Mot Prof Active Is Last"=FALSE, "Mot Prof Active Velocity Only"=FALSE, "Mot Prof Active Is Valid"=FALSE, "Mot Prof Buffer Is Full"=FALSE, "Mot Prof Active Profile Slot Select"=0, "Mot Prof NextID"=0, "Mot Prof Count"=0, "Mot Prof Active Velocity"=0.0, "Mot Prof Active Position"=0.0, "Mot Prof Output Enable"=0} ("Write After Receive"), "CAN Error"=w288, "Closed Loop Error"=w293, "Applied Throttle"=w301, "Module Enabled"=w311, "Reverse Limit Switch Closed"=w285, "Forward Limit Switch Closed"=w286) -> (w312:T2)
      n152 = Tick Count (ms)() -> (millisecond timer value=w287:u32)
      n153 = call <vilib>:"WPI_CANTalonSRX_Global.vi"("Write After Receive"=w312, "Operation"=WPI_CANTalonSRX_GlobalOps."Write After Receive General", "Device ID (0)"=w315) -> ()  [unwired: 6 in, 3 out]
    }
  }
  n154 = feedback-in #1(w18) -> ()
  "Device ID" <- "Device ID (0)"
